vi "Konvolucio MUDS150628 B232EATC Session SecurityAcess.vi"() -> ()   [LabVIEW 2011]
uses:
  <instrlib>/Konvolucio MUDS150628/Konvolucio MUDS150628.lvlib
panel:
  out "Key":string
  out "SeedByteArray":u8[](array[numeric]) format="%02x"
  out "SeedValue":u32 format="%08x"
  out "Seed":string
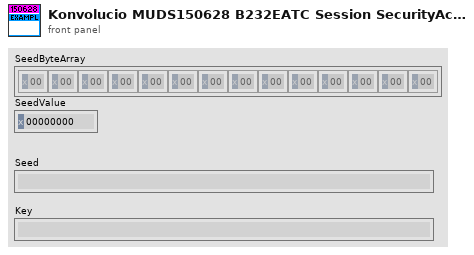
[diagram p1: front panel]
types:
  T1 = typedef "Konvolucio MUDS150628.lvlib/UdsHandleType.ctl" = cluster{"LogPath":path, "LogEnabled":bool, "isOpen":bool, "LogContent":string, "Adapter":string, "MCanHandle":T2, "TransmittId":u32, "ReceiveId":u32}
  T2 = typedef "Konvolucio MCAN120803.lvlib/MCanHandleType.ctl" = cluster{"MCanAdapter":refnum<k24>}
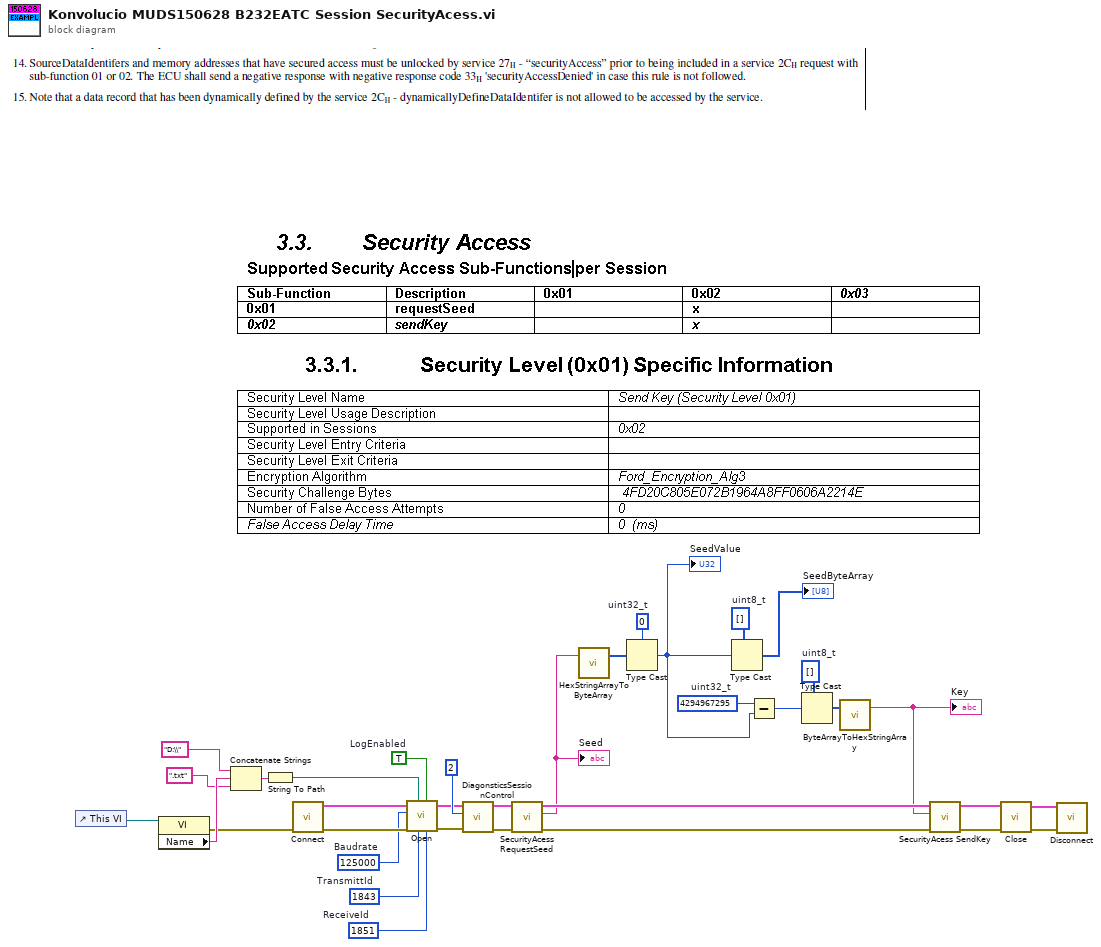
[diagram p0: block diagram]
diagram:
  w13 = TRUE  # LogEnabled
  w12 = u32 125000  # Baudrate
  w9 = u32 1851  # ReceiveId
  w10 = u32 1843  # TransmittId
  w23 = u8[] []  # uint8_t
  w25 = u32 4294967295  # uint32_t
  w27 = u8[] []  # uint8_t
  w28 = u32 0  # uint32_t
  n1 = control-ref of="This VI"() -> (w21:refnum<vi>)
  n2 = property class="VI"(reference=w21) -> (error out=w16:errorcluster, "Name"=w19:string)  [unwired: 1 in, 1 out]
  n3 = Concatenate Strings("D:\\" ("VI Name"), w19, ".txt" ("string")) -> (w17:string)
  n4 = String To Path(string=w17) -> (path=w11:path)
  n5 = call <instrlib>:"Connect.vi"("error in"=w16) -> ("error out"=w14:errorcluster, "UdsHandleOut"=w15:T1)  [unwired: 9 in]
  n6 = call <instrlib>:"Open.vi"("ReceiveId"=w9, "LogEnabled"=w13, "TransmittId"=w10, "LogPath"=w11, "error in"=w14, "BaudRate"=w12, "UdsHandleIn"=w15) -> ("error out"=w8:errorcluster, "UdsHandleOut"=w7:T1)  [unwired: 3 in]
  n7 = call <instrlib>:"DiagonsticsSessionControl.vi"("error in"=w8, "Session"=u8 2, "UdsHandleIn"=w7) -> ("error out"=w33:errorcluster, "UdsHandleOut"=w34:T1)  [unwired: 7 in]
  n8 = call <instrlib>:"SecurityAcess RequestSeed.vi"("error in"=w33, "UdsHandleIn"=w34) -> ("error out"=w29:errorcluster, "Seed"=w4:string, "UdsHandleOut"=w30:T1)  [unwired: 7 in]
  "Seed" <- w4
  n9 = call <instrlib>:"HexStringArrayToByteArray.vi"("HexStirngArray"=w4) -> ("ByteArrayOut"=w3:u8[])  [unwired: 2 in]
  n10 = Type Cast(type=w28, x=w3) -> (*(type *) &x=w24:u32)
  "SeedValue" <- w24
  n11 = Type Cast(type=w27, x=w24) -> (*(type *) &x=→"SeedByteArray":u8[])
  n12 = Subtract(x=w25, y=w24) -> (x-y=w22:u32)
  n13 = Type Cast(type=w23, x=w22) -> (*(type *) &x=w2:u8[])
  n14 = call <instrlib>:"ByteArrayToHexStringArray.vi"("ByteArrayIn"=w2) -> ("HexStringArrayOut"=w1:string)  [unwired: 2 in]
  "Key" <- w1
  n15 = call <instrlib>:"SecurityAcess SendKey.vi"("error in"=w29, "Key"=w1, "UdsHandleIn"=w30) -> ("error out"=w31:errorcluster, "UdsHandleOut"=w32:T1)  [unwired: 7 in]
  n16 = call <instrlib>:"Close.vi"("error in"=w31, "UdsHandleIn"=w32) -> ("error out"=w6:errorcluster, "UdsHandleOut"=w5:T1)  [unwired: 8 in]
  n17 = call <instrlib>:"Disconnect.vi"("error in"=w6, "UdsHandleIn"=w5) -> ()  [unwired: 9 in, 1 out]
